vi "subUpdateCSharpProjectFile.vi"(8 "error in (no error)":errorcluster, 11 ".csproj path":path) -> (0 "error out":errorcluster, 3 ".csproj path out":path)   [LabVIEW 2015, in "veristand-steps-codegen.lvlib"]
uses:
  veristand-steps-codegen.lvlib
  <vilib>/xml/Load XML File.vi
  <vilib>/xml/Close Reference(Node).vi
  <vilib>/xml/Close Reference(NNMap).vi
  <vilib>/ni/Simple XML/_polymorphics/Create Tag - Child with Text.vi
  <vilib>/xml/NI_XML.lvlib
  <resource>/objmgr/DOMUserDefRef.rc
  <vilib>/ni/Simple XML/Simple XML.lvlib
panel:
  out "error out":errorcluster
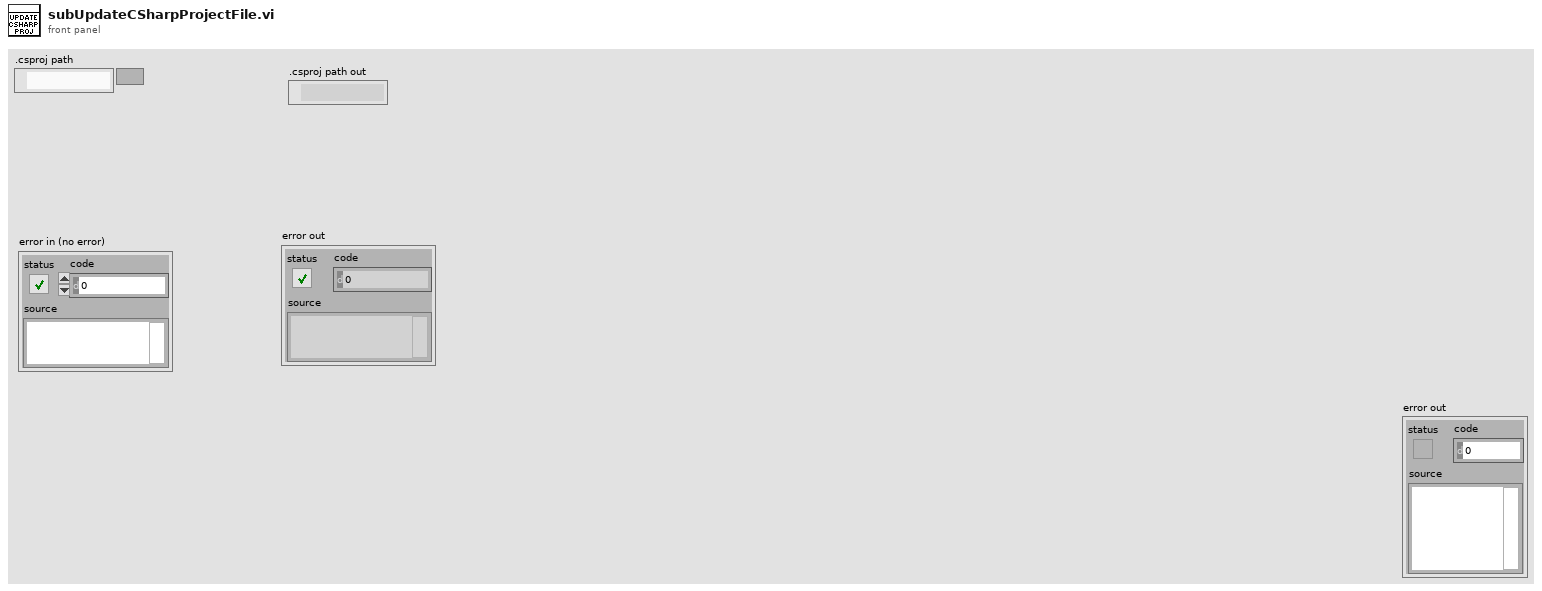
[diagram p1: front panel]
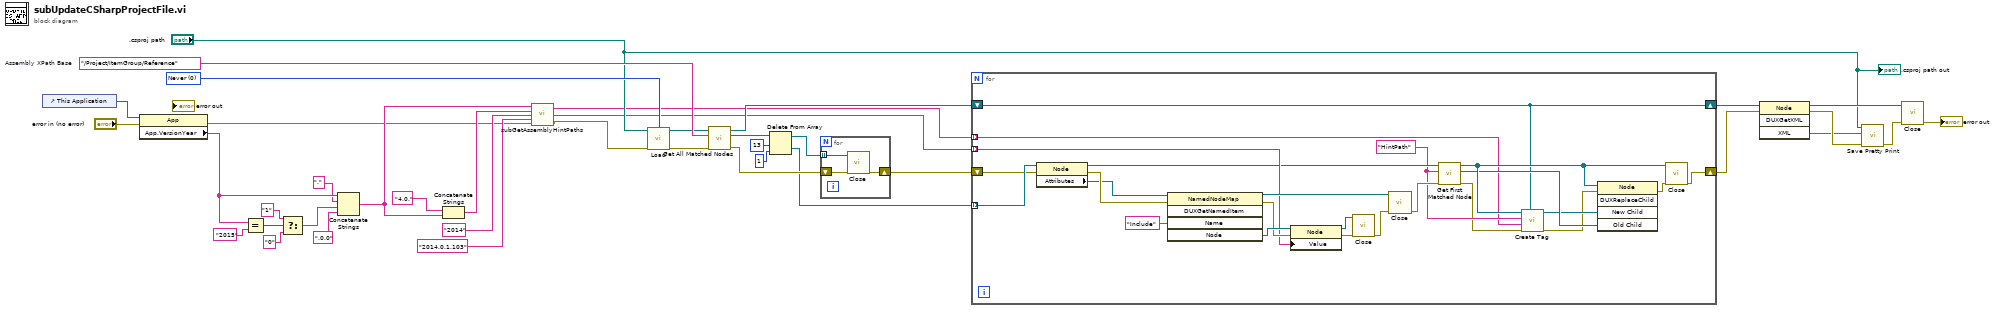
[diagram p0: block diagram]
diagram:
  w24 = "/Project/ItemGroup/Reference"  # Assembly XPath Base
  w21 = 0 items=["Never", "Always", "Auto"] ("validate on load (Auto)")
  n1 = control-ref of="This Application"() -> (w16:refnum<vi>)
  n2 = property class="App"(reference=w16, error in="error in (no error)") -> (error out=w2:errorcluster, "App.VersionYear"=w13:string)  [unwired: 1 out]
  n3 = Equal?(x=w13, y="2015") -> (x = y?=w11:bool)
  n4 = Select(t="1" ("string"), s=w11, f="0" ("string")) -> (s? t:f=w8:string)
  n5 = Concatenate Strings(w13, "." ("string"), w8, ".0.0" ("string")) -> (w5:string)
  n6 = Concatenate Strings("4.0." ("string"), w5) -> (w3:string)
  n7 = call "subGetAssemblyHintPaths.vi"("VeriStand assembly version string (2014.0.0.0)"=w5, "VeriStand GAC assembly version (4.0.2014.0.0.0)"=w3, "TestStand version string (2014)"="2014", "TestStand assembly version (2014.0.0.0)"="2014.0.1.103", "error in"=w2) -> ("New Assembly Hint Paths"=w17:string[], "New Assembly Include Paths"=w18:string[], "error out"=w19:errorcluster)  [unwired: 8 in]
  n8 = call-poly <vilib>:"Load.vi"("path to XML document"=".csproj path", "validate on load (Auto)"=w21, "error in (no error)"=w19) -> ("DOM document out"=w23:refnum<k20>, "error out"=w22:errorcluster)  [unwired: 10 in, 1 out]
  n9 = call <vilib>:"Get All Matched Nodes.vi"("error in (no error)"=w22, "XPath expression"=w24, "node in"=w23) -> ("error out"=w30:errorcluster, "node result array"=w25:refnum<k20>[], "node out"=w37:refnum<k20>)  [unwired: 6 in]
  n10 = Delete From Array(array=w25, length=13, index=1 ("length")) -> (deleted portion=w28:refnum<k20>[], array with subset deleted=w29:refnum<k20>[])
  n11 = for {
    tunnel: w29 -> [w42] mode=indexing
    shift-right: [w40] -> w31
    shift-left: w30 -> [w41]
    n12 = call-poly <vilib>:"Close.vi"("error in (no error)"=w41, "node"=w42) -> ("error out"=w40:errorcluster)  [unwired: 7 in]
  }
  n13 = for {
    tunnel: w28 -> [w63] mode=indexing
    shift-right: [w57] -> w32
    shift-left: w31 -> [w62]
    tunnel: w18 -> [w56] mode=indexing
    tunnel: w17 -> [w44] mode=indexing
    shift-right: [w43] -> w38
    shift-left: w37 -> [w43]
    w51 = "HintPath" ("XPath expression")
    n14 = property class="Node"(reference=w63, error in=w62) -> (reference out=w52:refnum<k20>, error out=w66:errorcluster, "Attributes"=w64:refnum<k20>)
    n15 = invoke class="NamedNodeMap" method="DUXGetNamedItem"(reference=w64, error in=w66, "Name"="Include") -> (reference out=w58:refnum<k20>, error out=w60:errorcluster, "Node"=w61:refnum<k20>)  [unwired: 2 in, 2 out]
    n16 = property class="Node"(reference=w61, error in=w60, "Value"=w56) -> (reference out=w59:refnum<k20>, error out=w55:errorcluster)
    n17 = call-poly <vilib>:"Close.vi"("error in (no error)"=w55, "node"=w59) -> ("error out"=w54:errorcluster)  [unwired: 7 in]
    n18 = call-poly <vilib>:"Close.vi"("error in (no error)"=w54, "named node map"=w58) -> ("error out"=w53:errorcluster)  [unwired: 7 in]
    n19 = call <vilib>:"Get First Matched Node.vi"("error in (no error)"=w53, "XPath expression"=w51, "node in"=w52) -> ("error out"=w50:errorcluster, "node result"=w48:refnum<k20>, "node out"=w49:refnum<k20>)  [unwired: 6 in]
    n20 = call-poly <vilib>:"Create Tag.vi"("DOM document reference"=w43, "error in (no error)"=w50, "Text Data"=w44, "Tag Name"=w51, "Parent Element reference"=w49) -> ("error out"=w46:errorcluster, "Child Element reference"=w47:refnum<k20>)  [unwired: 5 in]
    n21 = invoke class="Node" method="DUXReplaceChild"(reference=w49, error in=w46, "New Child"=w47, "Old Child"=w48) -> (error out=w45:errorcluster)  [unwired: 1 in, 4 out]
    n22 = call-poly <vilib>:"Close.vi"("error in (no error)"=w45, "node"=w49) -> ("error out"=w57:errorcluster)  [unwired: 7 in]
  }
  n23 = invoke class="Node" method="DUXGetXML"(reference=w38, error in=w32) -> (reference out=w36:refnum<k20>, error out=w34:errorcluster, "XML"=w33:string)  [unwired: 2 in, 1 out]
  n24 = call <vilib>:"Save Pretty Print.vi"("error in (no error)"=w34, "Pretty XML String"=w33, "XML file path"=".csproj path") -> ("error out"=w35:errorcluster)  [unwired: 7 in, 1 out]
  n25 = call-poly <vilib>:"Close.vi"("error in (no error)"=w35, "node"=w36) -> ("error out"=→"error out":errorcluster)  [unwired: 7 in]
  ".csproj path out" <- ".csproj path"
